vi "VISA shutter.vi"(8 "error in (no error)":errorcluster, 10 "button::shutter":bool, 11 "Cobolt in":refnum<class "Cobolt.lvclass">) -> (0 "error out":errorcluster, 3 "Cobolt out":refnum<class "Cobolt.lvclass">)   [LabVIEW 2012, in "Cobolt.lvclass"]
uses:
  Cobolt.lvclass
  Cobolt.lvclass/Cobolt.ctl
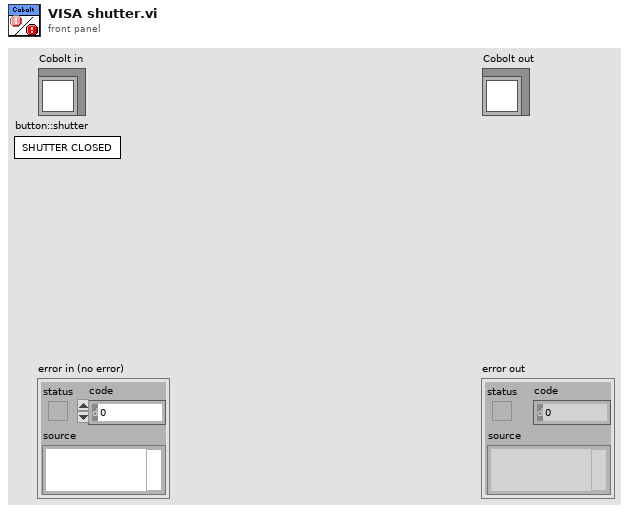
[diagram p1: front panel]
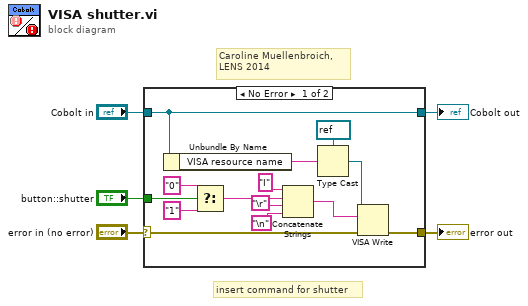
[diagram p0: block diagram]
diagram:
  # "Caroline Muellenbroich, \nLENS 2014"
  # "insert command for shutter"
  n1 = case shown="No Error" "error in (no error)" {
    selector: "error in (no error)" -> [w8 w21]
    tunnel: [w7 w21] -> w4
    tunnel: [w10 w20] -> w2
    tunnel: "Cobolt in" -> [w10 w20]
    tunnel: "button::shutter" -> [w9 _]
    frame No Error {
      n2 = Unbundle By Name(w10) -> ("VISA resource name"=w6:string)
      n3 = Select(t="0" ("string"), s=w9, f="1" ("string")) -> (s? t:f=w17:string)
      n4 = Concatenate Strings("I" ("string"), w17, "\r", "\n") -> (w18:string)
      n5 = Type Cast(type=refnum<visa-resource-name> refnum ("VISA resource name"), x=w6) -> (*(type *) &x=w14:refnum<visa-resource-name>)
      n6 = VISA Write(VISA resource name=w14, write buffer=w18, error in (no error)=w8) -> (error out=w7:errorcluster)  [unwired: 2 out]
    }
    frame Error {
    }
  }
  "error out" <- w4
  "Cobolt out" <- w2
